vi "PS35_SetStageAttributes.vi"(0 "Control unit ID":i32=1 min=1 max=10, 1 "Axis number":i32=1 min=1 max=3, 2 "Pitch":dbl=1.0 min=0.0001 step=0.1 format="%.4f", 3 "IncRev":i32=200 min=1, 4 "Ratio":dbl=1.0 min=0.0001 step=0.1 format="%.4f", 5 "error in (no error)":errorcluster) -> (19 "error out":errorcluster)   [LabVIEW 2020]
doc: "PS35_SetStageAttributes.vi, created: 06.03.2009 alex; last change: 22.10.2019 alex;\n\n<B>FUNCTION:</B> \n\nSet stage attributes for an axis.\nThe control unit uses for positioning of the axes internal values (increments).\nTo allow the positioning in other units (e.g., for linear measuring stages - mm,\nµm, for rotary measuring stages - degrees, mrad etc.), these parameters\nshould be defined. Then one is able to use the extended functions (...Ex) with\na desired unit. The specified values are converted internally into increments.\nThe movement of the slide per spindle revolution (pitch) is specified in a desired\nunit (e.g., 1 mm), as the first parameter for linear measuring stages. With the \nrotary measuring stages a revolution of the rotary table is specified in a desired\nunit (e.g., 360 degrees).\nThe number of the increments per motor revolution is defined as the second \nparameter. With the step motors it is the number of the full steps per revolution\n(e.g., 200). If a motor with the encoder is controlled, it is the number of the \nincrements per revolution (e.g., encoder with 4-fold evaluation: \nencoder lines number x 4 = 500x4).\nThe whole gear reduction ratio specified as the third parameter.\n----------------------------------------------------------------------------------------\n<B>INPUT:</B>\n[I32] <B>Control unit ID:</B> control unit index. (Default=1, Range=1...10) \n[I32] <B>Axis number:</B> axis number. (Default=1, Range=1...3) \n[DBL] <B>Pitch:</B> pitch. (Default=1.0) \n[I32] <B>IncRev:</B> pulses/steps per motor revolution. (Default=200) \n[DBL] <B>Ratio:</B> gear reduction ratio. (Default=1.0) \n[CLU] <B>error in</B>\n----------------------------------------------------------------------------------------\n<B>OUTPUT:</B>\n[CLU] <B>error out</B>\n----------------------------------------------------------------------------------------\n<B>SUB-VIs:</B>\n----------------------------------------------------------------------------------------\n<B>EXT-Calls:</B>\nps35.dll (V2.01)\n----------------------------------------------------------------------------------------"
uses:
  ps35.dll
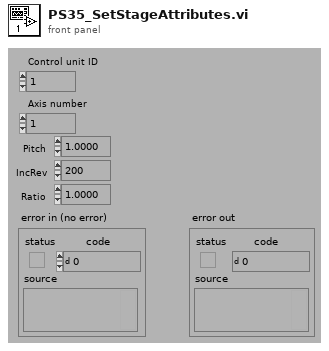
[diagram p1: front panel]
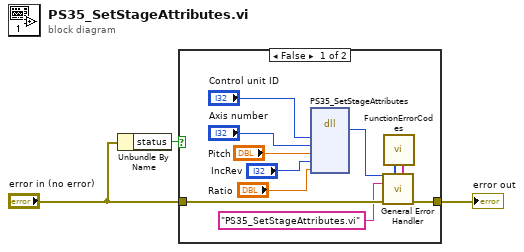
[diagram p0: block diagram]
diagram:
  n1 = Unbundle By Name("error in (no error)") -> ("status"=w1:bool)
  n2 = case shown="False" w1 {
    tunnel: "error in (no error)" -> [w13 w15]
    tunnel: [w12 w15] -> w3
    frame False {
      n3 = dll-call lib="C:/GEECS/Developers Version/source/Device Drivers/OwiSoft/OWISoftOEM/ps35/labview/lv82/ps35.dll" fn="PS35_SetStageAttributes" label="PS35_SetStage\nAttributes"("Index"="Control unit ID", "AxisNr"="Axis number", "Pitch"="Pitch", "IncRev"="IncRev", "Ratio"="Ratio") -> ("Rückgabetyp"=w11:i32)  [unwired: 8 in, 2 out]
      n4 = call "FunctionErrorCodes.vi"() -> ("[user-defined codes]"=w5:i32[], "[user-defined descriptions]"=w4:string[])  [unwired: 8 in]
      n5 = call <vilib>:"General Error Handler.vi"("[error code] (0)"=w11, "[user-defined codes]"=w5, "[user-defined descriptions]"=w4, "[error source] (\" \")"="PS35_SetStageAttributes.vi" ("[error source] (\" \")"), "error in (no error)"=w13) -> ("error out"=w12:errorcluster)  [unwired: 6 in, 4 out]
    }
    frame True {
    }
  }
  "error out" <- w3
